vi "Set VI Ref.vi"(1 "Instrument Prop In":T1 {"Private"."Offset" format="%^_3e"; "Private"."Scale Factors" format="%^_3e"}) -> (0 "Instrument Prop Out":T1 {"Private"."Offset" format="%^_3e"; "Private"."Scale Factors" format="%^_3e"})   [LabVIEW 2021]
uses:
  New NML Data Acq/Sub Controls/Instrument Properties.ctl
  New NML Data Acq/Sub Controls/Public.ctl
  New NML Data Acq/Sub Controls/Private.ctl
  New NML Data Acq/Sub Controls/Instrument Ref.ctl
  New NML Data Acq/Sub Controls/SystemCheckBox-resize.ctl
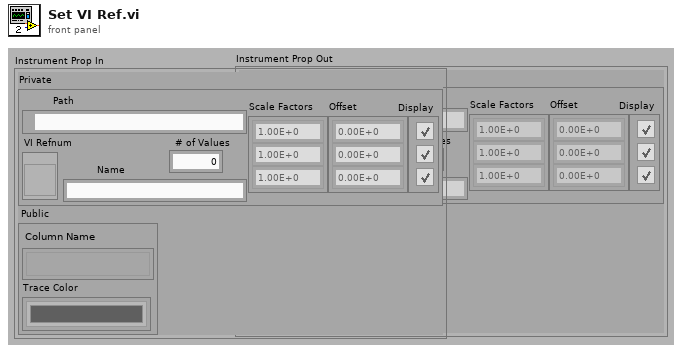
[diagram p1: front panel]
types:
  T1 = typedef "Instrument Properties.ctl" = cluster{"Public":T2, "Private":T3}
  T2 = typedef "Public.ctl" = cluster{"Column Name":string[], "Trace Color":u32[]}
  T3 = typedef "Private.ctl" = cluster{"Path":path, "VI Refnum":T4, "Name":string, "# of Values":i32, "Scale Factors":dbl[], "Display":T5[], "Offset":dbl[]}
  T4 = typedef "Instrument Ref.ctl" = refnum<vi>
  T5 = typedef "SystemCheckBox-resize.ctl" = bool
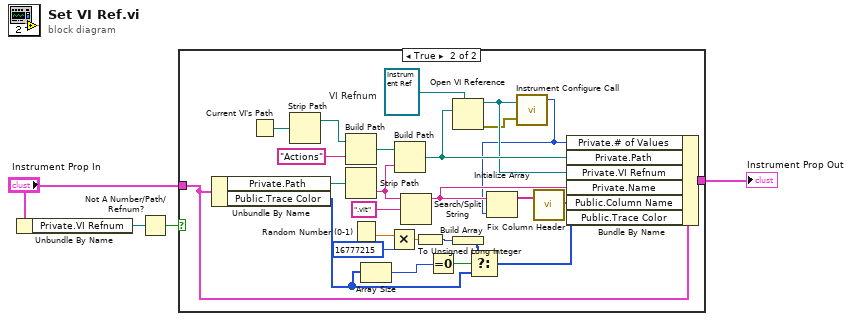
[diagram p0: block diagram]
diagram:
  n1 = Unbundle By Name("Instrument Prop In") -> ("Private.VI Refnum"=w2:T4)
  n2 = Not A Number/Path/Refnum?(number/path/refnum=w2) -> (NaN/Path/Refnum?=w1:bool)
  n3 = case shown="True" w1 {
    tunnel: "Instrument Prop In" -> [w5 w31]
    tunnel: [w5 w30] -> w3
    frame False {
    }
    frame True {
      w21 = T4 refnum  # VI Refnum
      n4 = Unbundle By Name(w31) -> ("Private.Path"=w24:path, "Public.Trace Color"=w9:u32[])
      n5 = Current VI's Path() -> (path=w29:path)
      n6 = Strip Path(path=w29) -> (stripped path=w25:path)  [unwired: 1 out]
      n7 = Build Path(base path=w25, name or relative path="Actions") -> (appended path=w27:path)
      n8 = Strip Path(path=w24) -> (name=w23:string)  [unwired: 1 out]
      n9 = Random Number (0-1)() -> (number: 0 to 1=w15:dbl)
      n10 = Array Size(array=w9) -> (size(s)=w10:i32)
      n11 = Multiply(x=w15, y=16777215) -> (x*y=w17:dbl)
      n12 = Build Path(base path=w27, name or relative path=w23) -> (appended path=w26:path)
      n13 = Search/Split String(string=w23, search string/char (-)=".vit") -> (substring before match=w7:string)  [unwired: 1 in, 2 out]
      n14 = To Unsigned Long Integer(number=w17) -> (unsigned 32bit integer=w13:u32)
      n15 = Equal To 0?(x=w10) -> (x = 0?=w14:bool)
      n16 = Open VI Reference(type specifier VI Refnum (for type only)=w21, vi path=w26) -> (vi reference=w20:T4, error out=w19:errorcluster)  [unwired: 4 in]
      n17 = Build Array(w13) -> (w11:u32[])
      n18 = Select(t=w11, s=w14, f=w9) -> (s? t:f=w12:u32[])
      n19 = call "Instrument Configure Call.vi"("VI Refnum"=w20, "error in"=w19) -> ("Numeric"=w6:i32)  [unwired: 2 out]
      n20 = Initialize Array(w7, w6) -> (w8:string[])
      n21 = call "Fix Column Header.vi"("Titles In"=w8) -> ("Titles Out"=w18:string[])  [unwired: 1 in]
      n22 = Bundle By Name(cluster=w31, "Private.# of Values"=w6, "Private.Path"=w26, "Private.VI Refnum"=w20, "Private.Name"=w7, "Public.Column Name"=w18, "Public.Trace Color"=w12) -> (w30:T1)
    }
  }
  "Instrument Prop Out" <- w3
